vi "Set Segments.vi"(8 "error in (no error)":errorcluster, 10 "Segments":string[](array[string]), 11 "URI in":refnum<class "URI.lvclass">) -> (0 "error out":errorcluster, 3 "URI out":refnum<class "URI.lvclass">)   [LabVIEW 2013, in "openURI.lvlib" / "URI.lvclass"]
uses:
  URI.lvclass
  URI.lvclass/URI.ctl
  components/path/Create Path (segments).vi
  checkCached.vi
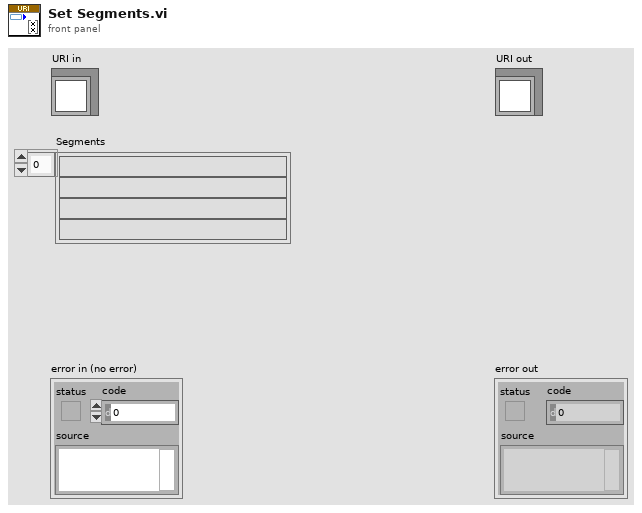
[diagram p1: front panel]
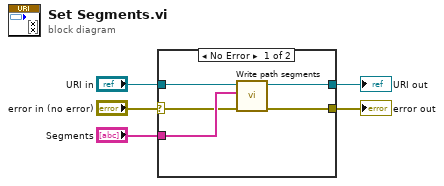
[diagram p0: block diagram]
diagram:
  n1 = case shown="No Error" "error in (no error)" {
    selector: "error in (no error)" -> [w7 w12]
    tunnel: [w6 w12] -> w4
    tunnel: [w8 w11] -> w2
    tunnel: "URI in" -> [w9 w11]
    tunnel: "Segments" -> [w10 _]
    frame No Error {
      n2 = call "Write path segments.vi"("error in (no error)"=w7, "Segments"=w10, "URI in"=w9) -> ("error out"=w6:errorcluster, "URI out"=w8:refnum<class "URI.lvclass">)  [unwired: 7 in]
    }
    frame Error {
    }
  }
  "error out" <- w4
  "URI out" <- w2
